vi "MessageCounter.vi"() -> (2 "Msg#":u32)   [LabVIEW 2021, in "YActor.lvclass"]
uses:
  YActor.lvclass
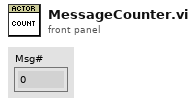
[diagram p1: front panel]
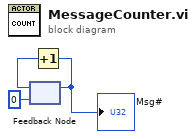
[diagram p0: block diagram]
diagram:
  n1 = feedback #1(u32 0) -> (w2:u32)
  n2 = Increment(x=w2) -> (x+1=w3:u32)
  "Msg#" <- w3
  n3 = feedback-in #1(w3) -> ()
